vi "nydybde.vi"() -> ()   [LabVIEW 2019]
uses:
  libRealSense3.lvlib
  <vilib>/ptbypt/NI_PtbyPt.lvlib
panel:
  out "Vel cam right leg":cluster{dbl, "Filtered x":dbl}(graph)
  in  "length 4":i32=100
  in  "index 4":i32=320
  in  "length 3":i32=140
  in  "index 3":i32=340
  out "Pos cam right leg":cluster{dbl, "Filtered x":dbl}(graph)
  out "Image 3":T1(plugin-control)
  in  "Image Type 3":T2 items=["Grayscale (U8)", "Grayscale (I16)", "Grayscale (SGL)", "Complex (CSG)", "RGB (U32)", "HSL (U32)", "RGB (U64)", "Grayscale (U16)"]
  in  "128 3":dbl=128.0 format="%#_13g"
  in  "Upper 3":dbl=2000.0 format="%#_13g"
  in  "Lower 3":dbl=500.0 format="%#_13g"
  in  "time 3":u32=100
  out "Vel cam left leg":cluster{dbl, "Filtered x":dbl}(graph)
  in  "length 2":i32=100
  in  "index 2":i32=220
  in  "length":i32=140
  in  "index":i32=340
  in  "time 2":u32=100
  out "Pos cam left leg":cluster{dbl, "Filtered x":dbl}(graph)
  out "Image 2":T1(plugin-control)
  in  "Image Type 2":T2 items=["Grayscale (U8)", "Grayscale (I16)", "Grayscale (SGL)", "Complex (CSG)", "RGB (U32)", "HSL (U32)", "RGB (U64)", "Grayscale (U16)"]
  in  "128 2":dbl=128.0 format="%#_13g"
  in  "Upper 2":dbl=2000.0 format="%#_13g"
  in  "Lower 2":dbl=500.0 format="%#_13g"
  out "Vel cam body":cluster{dbl, "Filtered x":dbl}(graph)
  out "Pos cam body":cluster{dbl, "Filtered x":dbl}(graph)
  in  "time 1":u32=100
  out "Image":T1(plugin-control)
  in  "Image Type":T2 items=["Grayscale (U8)", "Grayscale (I16)", "Grayscale (SGL)", "Complex (CSG)", "RGB (U32)", "HSL (U32)", "RGB (U64)", "Grayscale (U16)"]
  in  "128":dbl=128.0 format="%#_13g"
  in  "Upper":dbl=2000.0 format="%#_13g"
  in  "Lower":dbl=500.0 format="%#_13g"
  in  "y":dbl=2.0
  in  "Numeric 2":dbl=4.0 format="%#_13g"
  in  "Range Scale":enum16{"200m", "100m", "60m", "6m", "2m", "1m"}(ring)=enum."6m"
  in  "Device index":i32
  in  "Sensor index":i32
  in  "Select Depth \nResolution":u16(ring)=8 items=["256 x 144 @90fps", "480 x 270 @6fps", "480 x 270 @15fps", "480 x 270 @30fps", "480 x 270 @60fps", "640 x 360 @30fps", "640 x 480 @6fps", "640 x 480 @15fps", "640 x 480 @30fps", "848 x 480 @6fps", "848 x 480 @8fps", "848 x 480 @10fps", "1280 x 720 @6fps"]
  out "Depth map":sgl[][](graph)
  out "Numeric":i32
  out "Close Error":string="No Error\rNo Error\rNo Error\rNo Error"
  out "release frame error":string="No Error"
  out "Depth Capture":string="No Error"
  in  "stop":bool
  in  "laser on/off":bool
  in  "autoexposure":bool
  out "Config Error":string
  out "L-R Baseline, mm":sgl
  out "config error":string
  in  "Color Presets":T3(ring)=enum."D435"
  in  "Depth Presets":T4(ring)=enum."Face2"
  in  "Laser \nPower (mW)":dbl(slide)=155.72448 min=0.0 max=360.0 scale=0.36..360.0
  in  "Gain(16-248)":sgl=16.0 min=16 max=248
  in  "Exposure,us":sgl=33000.0
  out "Depth width":i32=1280
  out "Depth height":i32=720
  out "fx":sgl=656.61536 format="%#_5g"
  out "ppx":sgl=632.28015 format="%#_5g"
  out "fy":sgl=656.61536 format="%#_5g"
  out "ppy":sgl=357.01468 format="%#_5g"
  out "init error":string
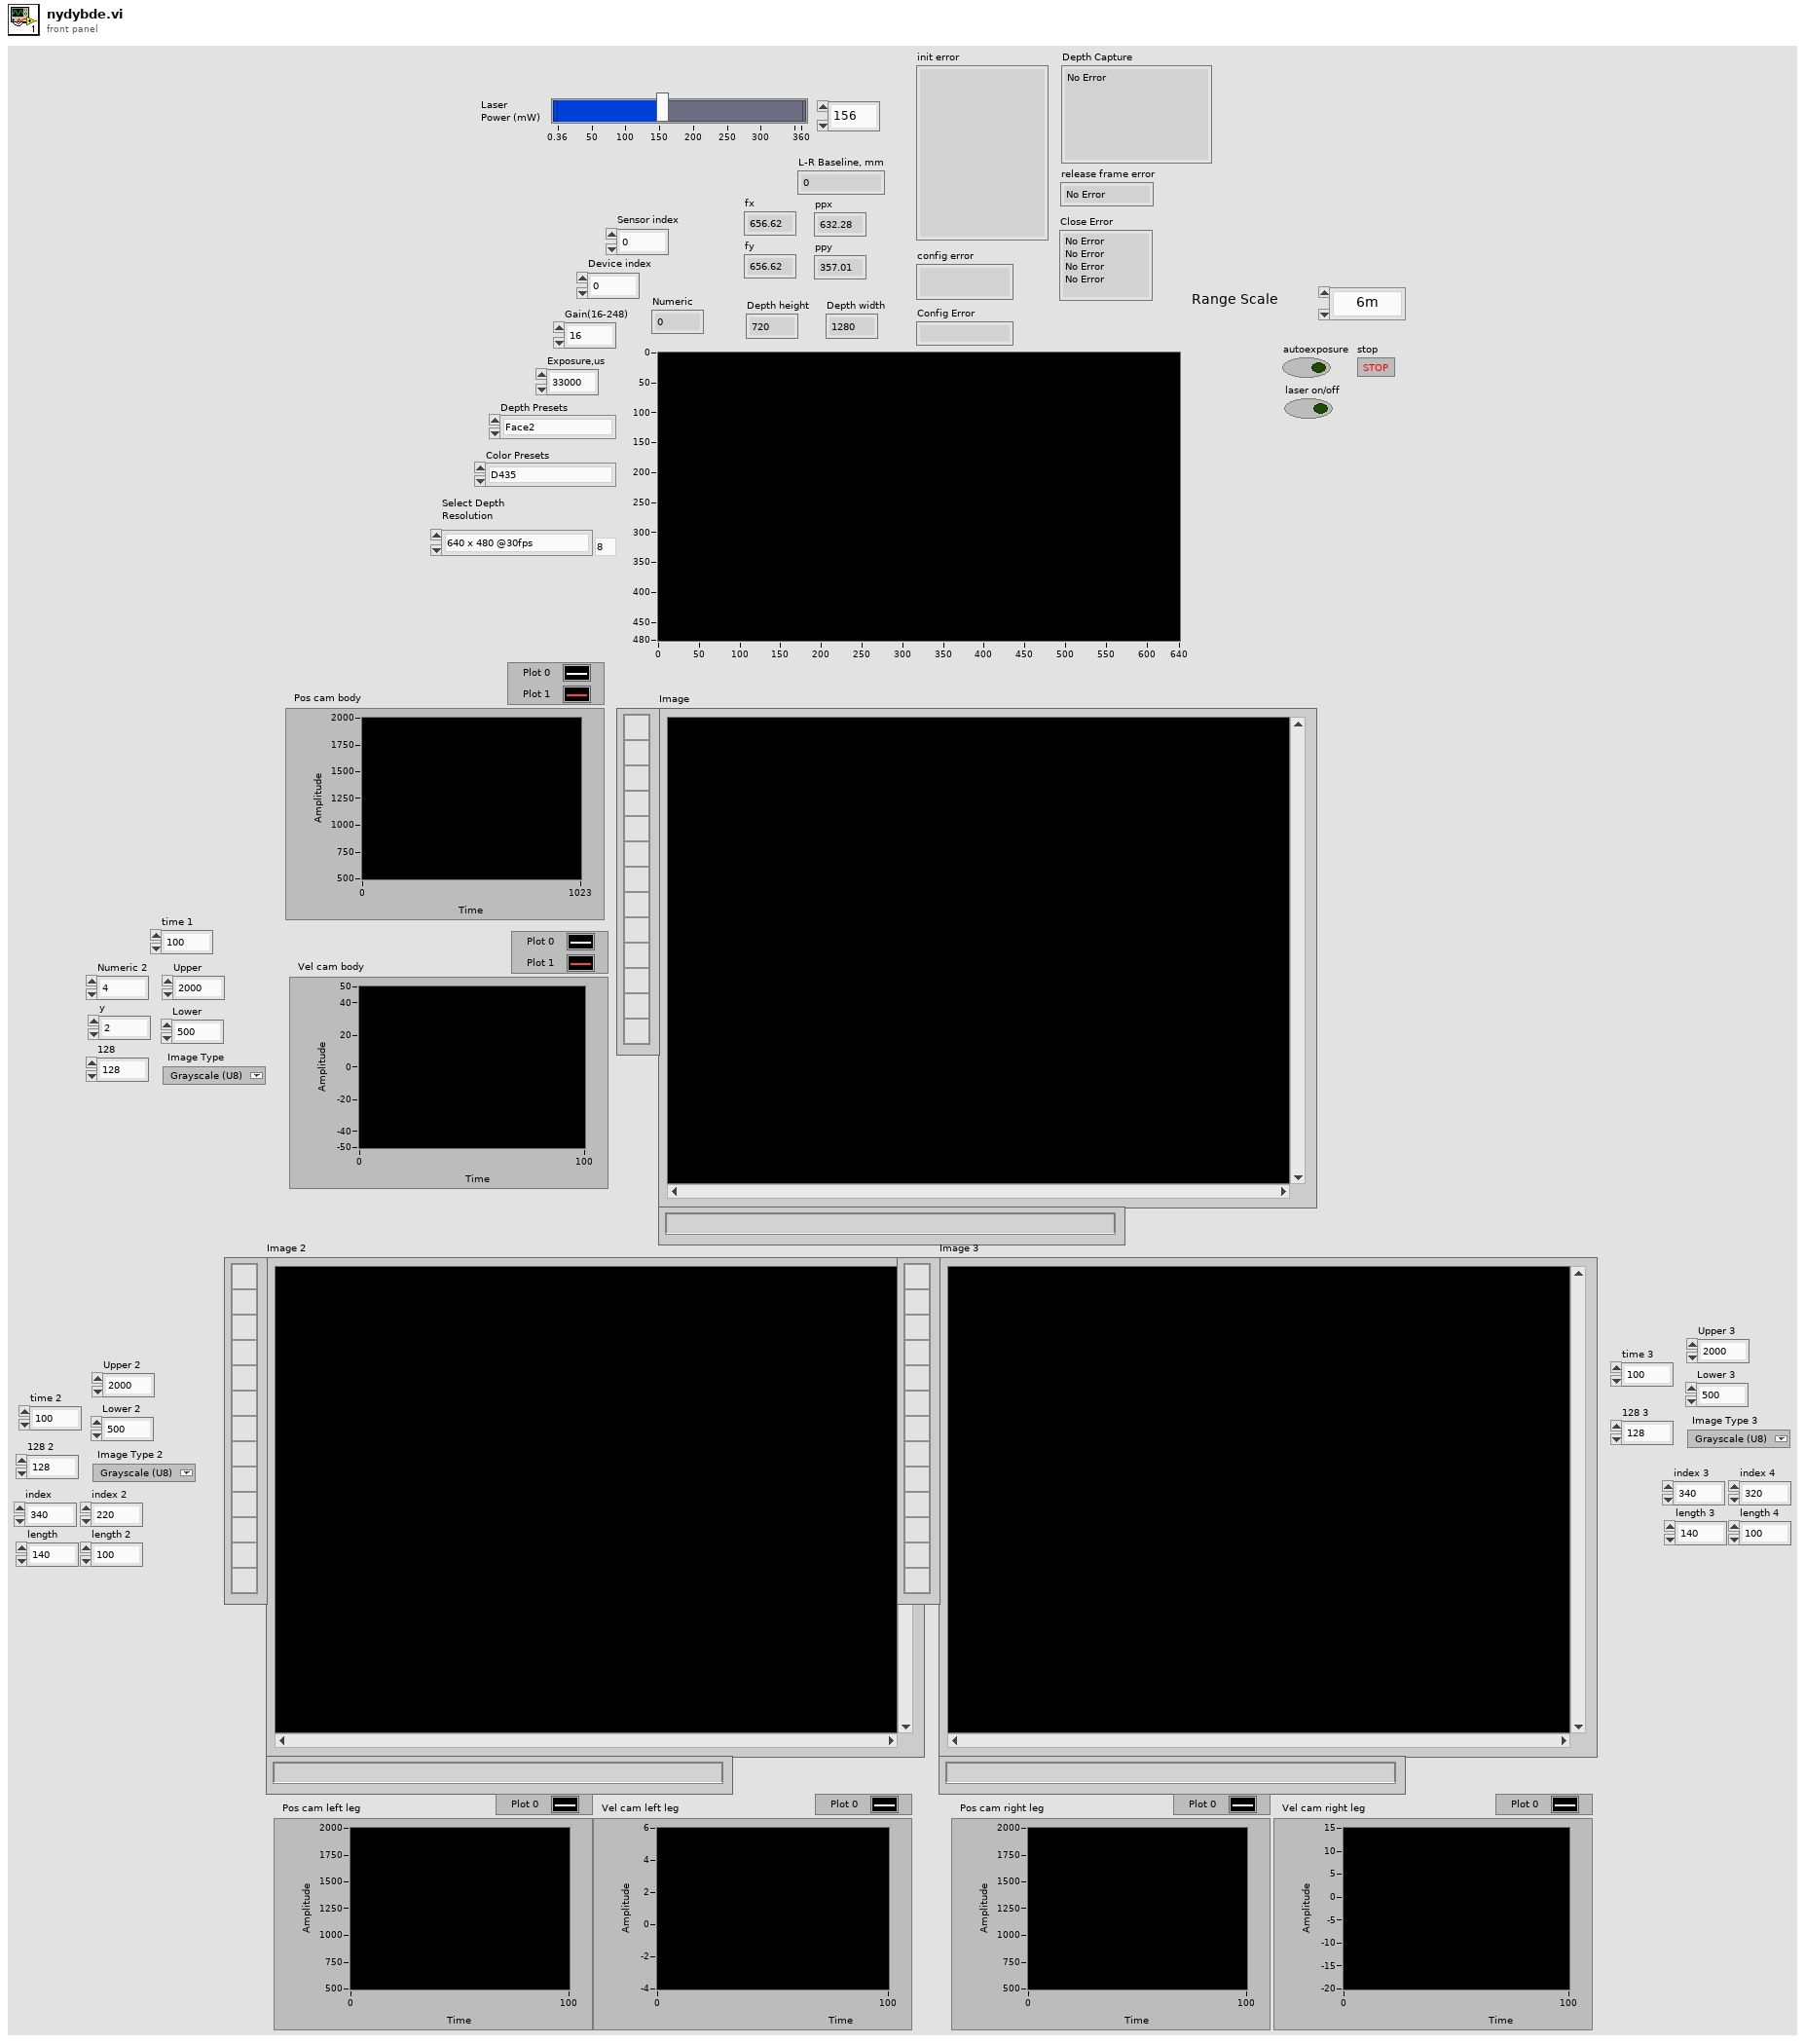
[diagram p1: front panel]
types:
  T1 = typedef "IMAQ Image.ctl" = refnum<image>
  T2 = typedef "Image Type" = u32
  T3 = enum16{"Custom", "RS400 (DS5p)", "RS400 (DS5p) 2", "RS400 (DS5p) 3", "RS400 (DS5p) 4", "RS400 (DS5p) 5", "RS410 (DS5a)", "RS410 (DS5a) 2", "DS410 (DS5a) 3", "DS410 (DS5a) 4", "DS410+IR", "DS5LR", "DS5LR-2", "DS5LR no pattern", "RS410 Remove IR", "RS410 Remove IR 2", "DS5micro", "D435"}
  T4 = enum16{"Custom", "Original", "New Depth 1", "New Depth 2", "Depth Active 1", "Active 3D Scan", "Active Short A", "Active Short C", "Face", "Face2", "Best Box", "High Density", "Medium Density", "High Accuracy", "Hand", "Short Range", "Flat wall", "Load .JSON", "Load .JSON2"}
  T5 = cluster{"camera name":string, "camera S/N":string, "F/W":string, "Sensor name":string, "api_version":i32, "rscontext":u64, "device_list":u64, "device count":i32, "Dev out":u64, "sensor_list":u64, "sensor count":i32, "Sensor out":u64}
  T6 = cluster{"width":i32, "height":i32, "fps":i32, "Profile":u64, "ppx":sgl, "ppy":sgl, "fx":sgl, "fy":sgl, "model":u32}
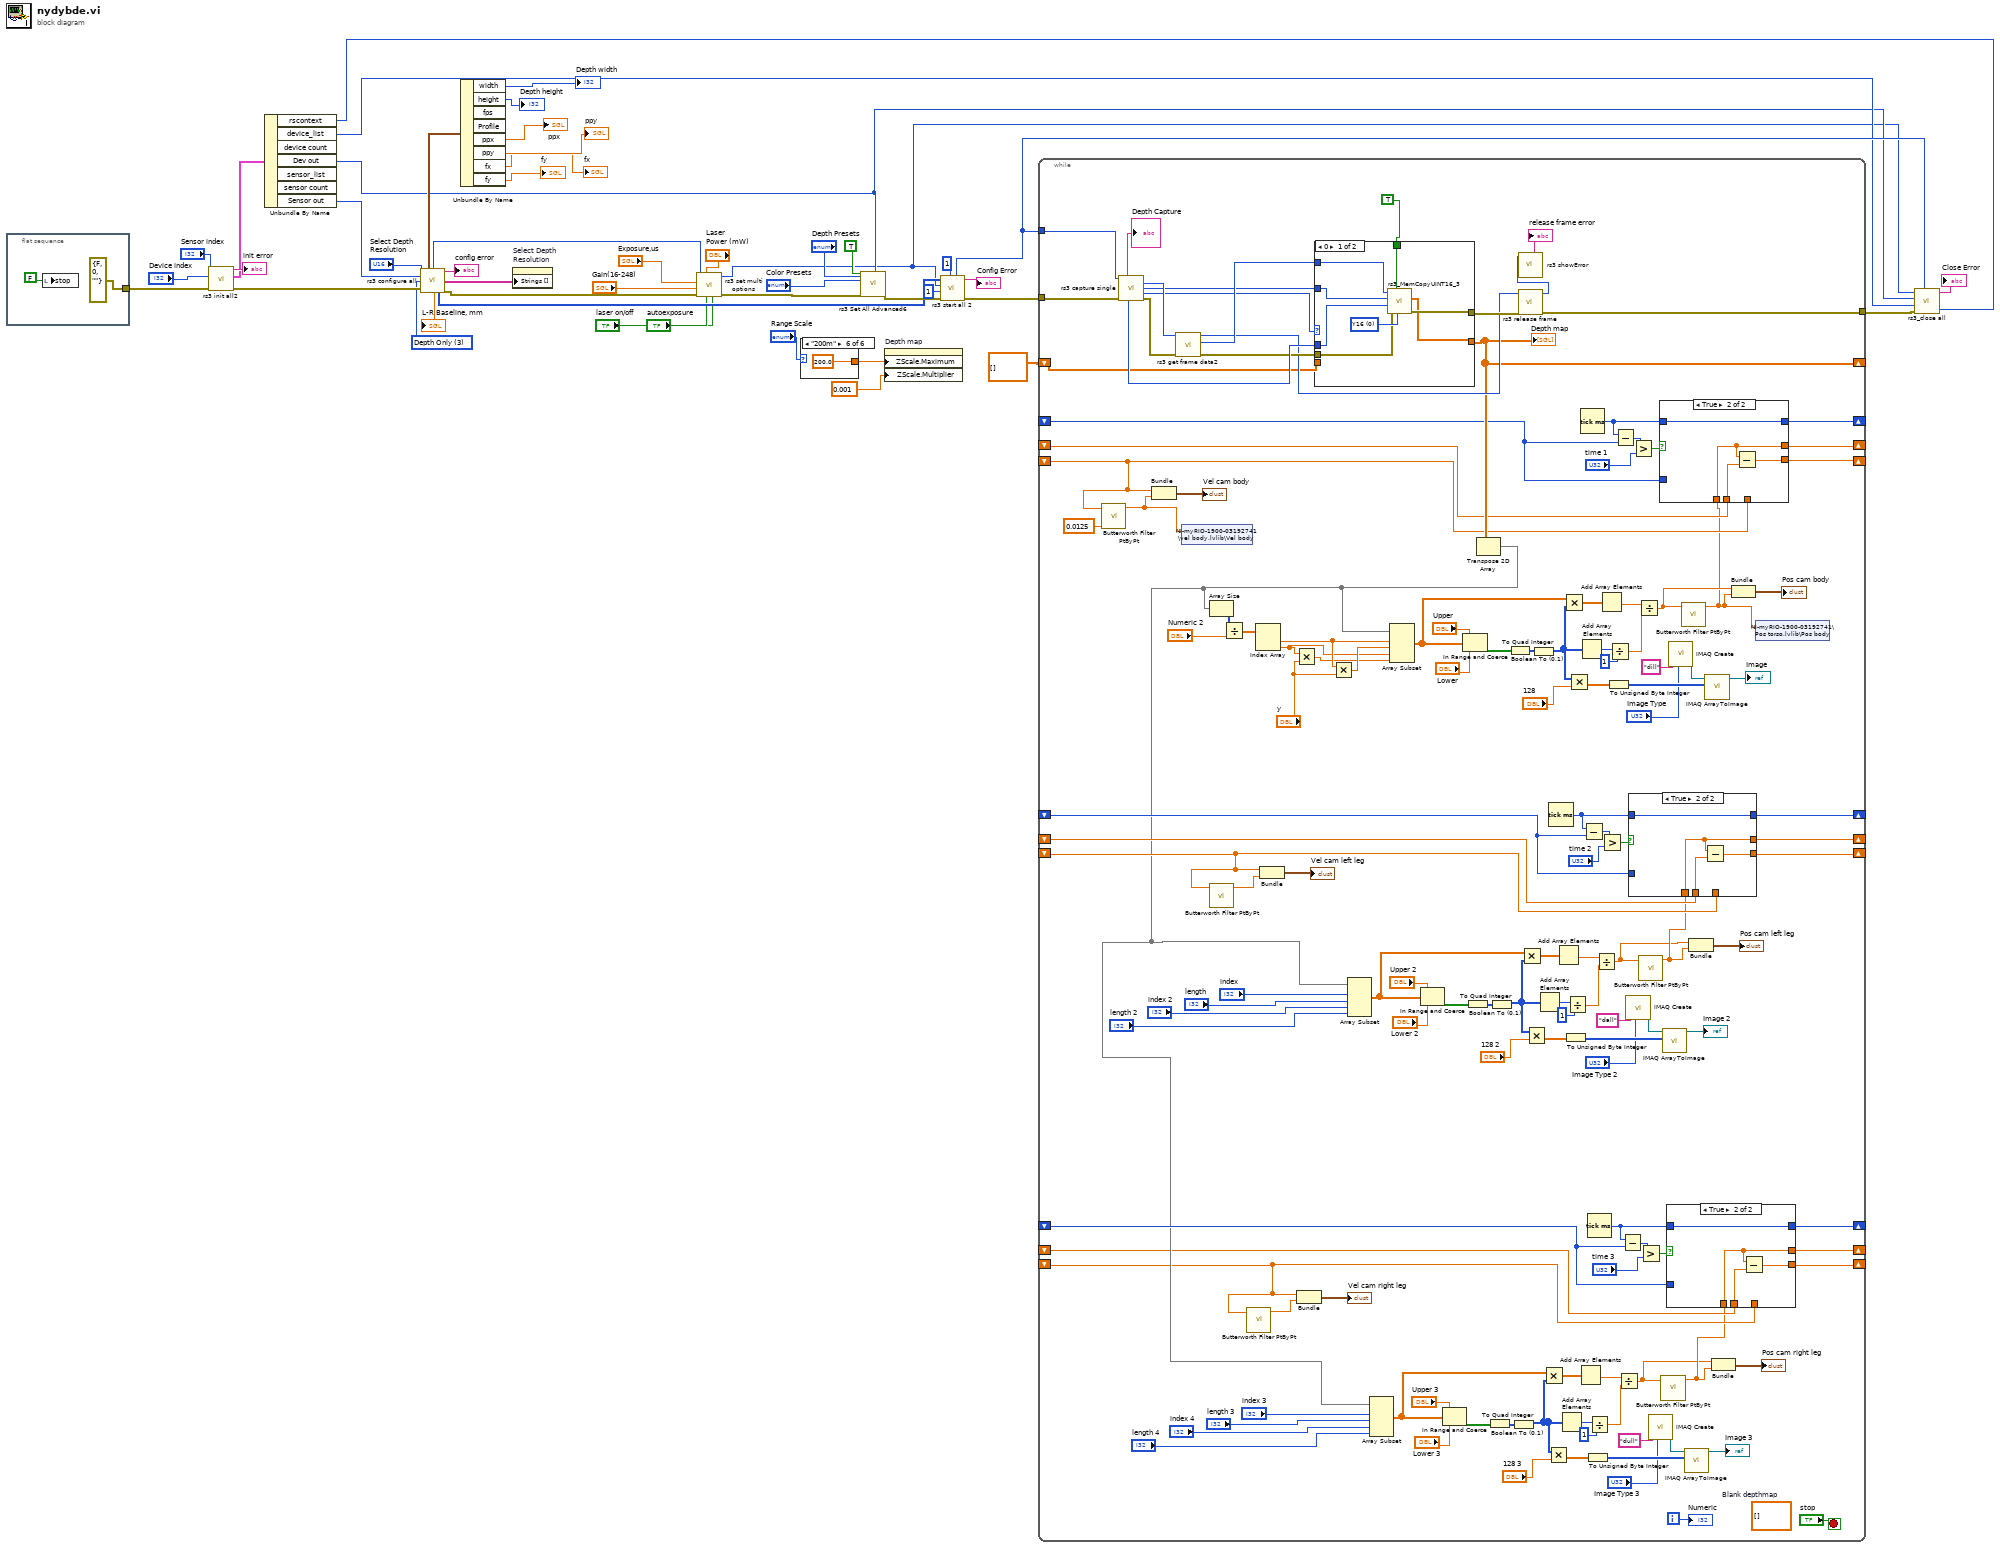
[diagram p0: block diagram]
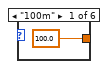
[diagram p2: hidden frame]
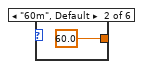
[diagram p3: hidden frame]
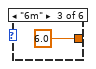
[diagram p4: hidden frame]
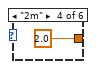
[diagram p5: hidden frame]
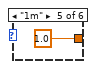
[diagram p6: hidden frame]
diagram:
  w8 = u16 3 items=["Depth + Left Color", "Unrectified L + R", "Rectified L + R", "Depth Only", "RGB ext. Only"] ("Stream selection")
  n1 = flat-sequence {
    tunnel: [errorcluster {"status"=FALSE, "code"=0, "source"=""} ("error in")] -> w28
    frame #0 {
      n2 = local write "stop"(FALSE) -> ()
    }
  }
  n3 = call "rs3 init all2.vi"("error in"=w28, "Select Device"="Device index", "Select Sensor"="Sensor index") -> ("error out"=w46:errorcluster, "init results"=w14:T5, "init error"=→"init error":string)  [unwired: 2 in, 4 out]
  n4 = Unbundle By Name(w14) -> ("rscontext"=w11:u64, "device_list"=w12:u64, "Dev out"=w10:u64, "Sensor out"=w13:u64)  [unwired: 3 out]
  n5 = call "rs3 configure all.vi"("Select Resolution"="Select Depth \nResolution", "Sensor in"=w13, "Stream selection"=w8, "error in (no error)"=w46) -> ("Output stream L"=w38:T6, "Sensor out"=w23:u64, "config error"=→"config error":string, "Output stream"=w45:string[], "L-R Baseline, mm"=→"L-R Baseline, mm":sgl, "Stream Profile Handles"=w25:u64[], "error out"=w35:errorcluster)  [unwired: 2 in, 3 out]
  n6 = Unbundle By Name(w38) -> ("width"=→"Depth width":i32, "height"=→"Depth height":i32, "ppx"=→"ppx":sgl, "ppy"=→"ppy":sgl, "fx"=→"fx":sgl, "fy"=→"fy":sgl)  [unwired: 2 out]
  n7 = property on="Select Depth \nResolution" class="Ring (strict)"("Strings []"=w45) -> ()  [unwired: 2 in, 2 out]
  n8 = call "rs3 set multi options.vi"("laser on/off"="laser on/off", "autoexposure"="autoexposure", "Laser power, mW (0-360)"="Laser \nPower (mW)", "error in (no error)"=w35, "Gain(16-248)"="Gain(16-248)", "Exposure, us"="Exposure,us", "Sensor in"=w23) -> ("error out"=w30:errorcluster, "Sensor out"=w9:u64)  [unwired: 2 in, 1 out]
  n9 = case shown="\"200m\"" "Range Scale" {
    tunnel: [100.0 ("Z Scale.Offset and Multiplier:Multiplier") 60.0 ("Z Scale.Offset and Multiplier:Multiplier") 6.0 ("Z Scale.Offset and Multiplier:Multiplier") 2.0 ("Z Scale.Offset and Multiplier:Multiplier") 1.0 ("Z Scale.Offset and Multiplier:Multiplier") 200.0 ("Z Scale.Offset and Multiplier:Multiplier")] -> w2
    frame "100m" {
    }
    frame "60m", Default {
    }
    frame "6m" {
    }
    frame "2m" {
    }
    frame "1m" {
    }
    frame "200m" {
    }
  }
  n10 = call "rs3 Set All Advanced6.vi"("Set Color Corr"=TRUE, "Depth Presets"="Depth Presets", "Color Presets"="Color Presets", "error in (no error)"=w30, "device in"=w10) -> ("error out"=w29:errorcluster)  [unwired: 20 in, 2 out]
  n11 = property on="Depth map" class="IntGraph (strict)"("ZScale.Maximum"=w2, "ZScale.Multiplier"=0.001 ("Z Scale.Offset and Multiplier:Multiplier")) -> ()  [unwired: 2 in, 2 out]
  n12 = call "rs3 start all 2.vi"("capacity"=1, "error in (no error)"=w29, "Count of Streams"=1, "Sensor in"=w9, "Stream profile array"=w25) -> ("error out"=w18:errorcluster, "Config Error"=→"Config Error":string, "queue out"=w15:u64)  [unwired: 3 in, 1 out]
  n13 = while {
    tunnel: w15 -> [w188]
    tunnel: w18 -> [w187]
    tunnel: [w177] -> w16
    shift-right: [w173] -> _
    shift-left: sgl[][] [] ("2D Array Output") -> [w174]
    shift-right: [w146] -> _
    shift-left: _ -> [w144]
    shift-right: [w140] -> _
    shift-left: _ -> [w139]
    shift-right: [w138] -> _
    shift-left: _ -> [w136]
    shift-right: [w112] -> _
    shift-left: _ -> [w111]
    shift-right: [w109] -> _
    shift-left: _ -> [w101]
    shift-right: [w110] -> _
    shift-left: _ -> [w108]
    shift-right: [w96] -> _
    shift-left: _ -> [w95]
    shift-right: [w70] -> _
    shift-left: _ -> [w69]
    shift-right: [w68] -> _
    shift-left: _ -> [w65]
    i -> [w175]
    stop <- "stop" stop-if-true
    (unwired) sgl[][] []  # Blank depthmap
    n14 = call <vilib>:"Butterworth Filter PtByPt.vi"("low cutoff freq: fl"=0.0125, "x"=w136) -> ("Filtered x"=w57:dbl)  [unwired: 7 in, 1 out]
    n15 = call "rs3 capture single.vi"("queue in"=w188, "error in (no error)"=w187) -> ("Capture Error"=→"Depth Capture":string, "frame out"=w190:u64, "width"=w185:i32, "Stream type"=w182:u16, "height"=w184:i32, "error out"=w189:errorcluster)  [unwired: 5 in, 3 out]
    n16 = Bundle(w136, "Filtered x"=w57) -> (→"Vel cam body":cluster{dbl, "Filtered x":dbl})  [unwired: 1 in]
    n17 = call "rs3 get frame data2.vi"("error in (no error)"=w189, "frame in"=w190) -> ("error out"=w183:errorcluster, "image pointer out"=w186:u64, "Frame out"=w176:u64)  [unwired: 6 in, 1 out]
    n18 = shared-variable "NI-myRIO-1900-03192741\\vel body.lvlib\\Vel body"(w57) -> ()  [unwired: 1 in, 1 out]
    n19 = call <vilib>:"Butterworth Filter PtByPt.vi"("x"=w101) -> ("Filtered x"=w102:dbl)  [unwired: 8 in, 1 out]
    n20 = call <vilib>:"Butterworth Filter PtByPt.vi"("x"=w65) -> ("Filtered x"=w66:dbl)  [unwired: 8 in, 1 out]
    n21 = Bundle(w101, "Filtered x"=w102) -> (→"Vel cam left leg":cluster{dbl, "Filtered x":dbl})  [unwired: 1 in]
    n22 = Bundle(w65, "Filtered x"=w66) -> (→"Vel cam right leg":cluster{dbl, "Filtered x":dbl})  [unwired: 1 in]
    n23 = case shown="0" w182 {
      tunnel: w186 -> [w214 _]
      tunnel: w185 -> [w218 _]
      tunnel: w184 -> [w219 _]
      tunnel: w183 -> [w220 w223]
      tunnel: [w217 w223] -> w178
      tunnel: [w216 w222] -> w173
      tunnel: TRUE -> [w215 _]
      tunnel: w174 -> [_ w222]
      frame 0 {
        w221 = u16 0 items=["Y16", "Y8"] ("Image format")
        n24 = call "rs3_MemCopyUINT16_3.vi"("Image format"=w221, "Transpose"=w215, "error in (no error)"=w220, "Depth Y"=w219, "Depth X"=w218, "Zimage pointer"=w214) -> ("error out"=w217:errorcluster, "2D Array Output"=w216:sgl[][])  [unwired: 2 in, 2 out]
      }
      frame 1, Default {
      }
    }
    "Depth map" <- w173
    n25 = Transpose 2D Array(2D array=w173) -> (transposed array=w71:sgl[][])
    n26 = Array Size(array=w71) -> (size(s)=w172:i32[])
    n27 = Divide(x=w172, y="Numeric 2") -> (x/y=w170:dbl[])
    n28 = Index Array(array=w170) -> (element #1=w169:dbl, element #2=w165:dbl)  [unwired: 2 in]
    n29 = Multiply(x=w165, y="y") -> (x*y=w166:dbl)
    n30 = Multiply(x=w169, y="y") -> (x*y=w168:dbl)
    n31 = Array Subset(array=w71, index (row)="index", length (row)="length", index (col)="index 2", length (col)="length 2") -> (w129:sgl[][])
    n32 = Array Subset(array=w71, index (row)="index 3", length (row)="length 3", index (col)="index 4", length (col)="length 4") -> (w88:sgl[][])
    n33 = Array Subset(array=w71, index (row)=w169, length (row)=w168, index (col)=w165, length (col)=w166) -> (w158:sgl[][])
    n34 = In Range and Coerce(upper limit="Upper 2", x=w129, lower limit="Lower 2") -> (In Range?=w133:bool[][])  [unwired: 1 out]
    n35 = In Range and Coerce(upper limit="Upper 3", x=w88, lower limit="Lower 3") -> (In Range?=w92:bool[][])  [unwired: 1 out]
    n36 = In Range and Coerce(upper limit="Upper", x=w158, lower limit="Lower") -> (In Range?=w162:bool[][])  [unwired: 1 out]
    n37 = Boolean To (0,1)(Boolean=w133) -> (0, 1=w132:i16[][])
    n38 = Boolean To (0,1)(Boolean=w92) -> (0, 1=w91:i16[][])
    n39 = To Quad Integer(1:w132) -> (0:w128:i64[][])
    n40 = Boolean To (0,1)(Boolean=w162) -> (0, 1=w161:i16[][])
    n41 = To Quad Integer(1:w91) -> (0:w87:i64[][])
    n42 = call "rs3 release frame.vi"("error in (no error)"=w178, "Frame"=w176) -> ("error out"=w177:errorcluster, "error"=w179:u64)  [unwired: 8 in]
    n43 = call "rs3 showError.vi"("error"=w179) -> ("Error summary"=→"release frame error":string)  [unwired: 6 in, 4 out]
    n44 = Multiply(x=w129, y=w128) -> (x*y=w131:sgl[][])
    n45 = Multiply(x=w128, y="128 2") -> (x*y=w123:dbl[][])
    n46 = To Quad Integer(1:w161) -> (0:w157:i64[][])
    n47 = Add Array Elements(numeric array=w128) -> (sum=w127:i64)
    n48 = Multiply(x=w88, y=w87) -> (x*y=w90:sgl[][])
    n49 = Multiply(x=w87, y="128 3") -> (x*y=w82:dbl[][])
    n50 = Tick Count (ms)() -> (millisecond timer value=w116:u32)
    n51 = Add Array Elements(numeric array=w131) -> (sum=w124:sgl)
    n52 = Add Array Elements(numeric array=w87) -> (sum=w86:i64)
    n53 = Multiply(x=w158, y=w157) -> (x*y=w160:sgl[][])
    n54 = To Unsigned Byte Integer(number=w123) -> (unsigned 8bit integer=w122:u8[][])
    n55 = Divide(x=w127, y=i64 1) -> (x/y=w125:dbl)
    n56 = Multiply(x=w157, y="128") -> (x*y=w152:dbl[][])
    n57 = Add Array Elements(numeric array=w90) -> (sum=w83:sgl)
    n58 = Add Array Elements(numeric array=w157) -> (sum=w156:i64)
    n59 = Tick Count (ms)() -> (millisecond timer value=w145:u32)
    n60 = Subtract(x=w116, y=w111) -> (x-y=w114:u32)
    n61 = To Unsigned Byte Integer(number=w82) -> (unsigned 8bit integer=w81:u8[][])
    n62 = Tick Count (ms)() -> (millisecond timer value=w100:u32)
    n63 = Divide(x=w86, y=i64 1) -> (x/y=w84:dbl)
    n64 = Divide(x=w124, y=w125) -> (x/y=w60:dbl)
    n65 = Add Array Elements(numeric array=w160) -> (sum=w153:sgl)
    n66 = Greater?(x=w114, y="time 2") -> (0:w115:bool)
    n67 = To Unsigned Byte Integer(number=w152) -> (unsigned 8bit integer=w151:u8[][])
    n68 = Divide(x=w156, y=i64 1) -> (x/y=w154:dbl)
    n69 = Subtract(x=w145, y=w144) -> (x-y=w142:u32)
    n70 = Divide(x=w83, y=w84) -> (x/y=w59:dbl)
    n71 = Subtract(x=w100, y=w95) -> (x-y=w98:u32)
    n72 = call "IMAQ Create"("Image Name"="dall", "Image Type"="Image Type 2") -> ("New Image"=w121:T1)  [unwired: 3 in, 1 out]
    n73 = Greater?(x=w142, y="time 1") -> (0:w143:bool)
    n74 = Divide(x=w153, y=w154) -> (x/y=w61:dbl)
    n75 = call <vilib>:"Butterworth Filter PtByPt.vi"("x"=w60) -> ("Filtered x"=w64:dbl)  [unwired: 8 in, 1 out]
    n76 = case shown="True" w115 {
      tunnel: w116 -> [_ w206]
      tunnel: [w202 w206] -> w112
      tunnel: w111 -> [w202 _]
      tunnel: w64 -> [_ w205]
      tunnel: [w201 w205] -> w110
      tunnel: w108 -> [w201 w204]
      tunnel: [w200 w203] -> w109
      tunnel: w101 -> [w200 _]
      frame False {
      }
      frame True {
        n77 = Subtract(x=w205, y=w204) -> (x-y=w203:dbl)
      }
    }
    n78 = Greater?(x=w98, y="time 3") -> (0:w99:bool)
    n79 = call "IMAQ Create"("Image Name"="dull", "Image Type"="Image Type 3") -> ("New Image"=w80:T1)  [unwired: 3 in, 1 out]
    n80 = call <vilib>:"Butterworth Filter PtByPt.vi"("x"=w59) -> ("Filtered x"=w63:dbl)  [unwired: 8 in, 1 out]
    n81 = call "IMAQ ArrayToImage"("Image Pixels (U8)"=w122, "Image"=w121) -> ("Image Out"=→"Image 2":T1)  [unwired: 8 in, 1 out]
    n82 = case shown="True" w99 {
      tunnel: w100 -> [_ w199]
      tunnel: [w195 w199] -> w96
      tunnel: w95 -> [w195 _]
      tunnel: w63 -> [_ w198]
      tunnel: [w194 w198] -> w70
      tunnel: w69 -> [w194 w197]
      tunnel: [w193 w196] -> w68
      tunnel: w65 -> [w193 _]
      frame False {
      }
      frame True {
        n83 = Subtract(x=w198, y=w197) -> (x-y=w196:dbl)
      }
    }
    n84 = call "IMAQ Create"("Image Name"="dill", "Image Type"="Image Type") -> ("New Image"=w150:T1)  [unwired: 3 in, 1 out]
    n85 = call <vilib>:"Butterworth Filter PtByPt.vi"("x"=w61) -> ("Filtered x"=w58:dbl)  [unwired: 8 in, 1 out]
    n86 = case shown="True" w143 {
      tunnel: w145 -> [_ w213]
      tunnel: [w209 w213] -> w146
      tunnel: w144 -> [w209 _]
      tunnel: w58 -> [_ w212]
      tunnel: [w208 w212] -> w140
      tunnel: w139 -> [w208 w211]
      tunnel: [w207 w210] -> w138
      tunnel: w136 -> [w207 _]
      frame False {
      }
      frame True {
        n87 = Subtract(x=w212, y=w211) -> (x-y=w210:dbl)
      }
    }
    n88 = call "IMAQ ArrayToImage"("Image Pixels (U8)"=w81, "Image"=w80) -> ("Image Out"=→"Image 3":T1)  [unwired: 8 in, 1 out]
    n89 = Bundle(w60, "Filtered x"=w64) -> (→"Pos cam left leg":cluster{dbl, "Filtered x":dbl})  [unwired: 1 in]
    n90 = call "IMAQ ArrayToImage"("Image Pixels (U8)"=w151, "Image"=w150) -> ("Image Out"=→"Image":T1)  [unwired: 8 in, 1 out]
    n91 = Bundle(w59, "Filtered x"=w63) -> (→"Pos cam right leg":cluster{dbl, "Filtered x":dbl})  [unwired: 1 in]
    n92 = Bundle(w61, "Filtered x"=w58) -> (→"Pos cam body":cluster{dbl, "Filtered x":dbl})  [unwired: 1 in]
    n93 = shared-variable "NI-myRIO-1900-03192741\\Pos torso.lvlib\\Pos body"(w58) -> ()  [unwired: 1 in, 1 out]
    "Numeric" <- w175
  }
  n94 = call "rs3_close all.vi"("rscontext"=w11, "queue in"=w15, "error in (no error)"=w16, "device_list"=w12, "Dev in"=w10, "Sensor in"=w9) -> ("Close Error"=→"Close Error":string)  [unwired: 4 in, 1 out]
